vi "Initialize PID Parameters Channel Browsers.vi"(6 "Enable Gain Scheduling":bool, 8 "error in (no error)":errorcluster, 10 "Channel Browser":refnum<k24>, 11 "Item Ref in":T2 format="%.0x") -> (0 "error out":errorcluster, 2 "Refs":T1, 3 "Item Ref out":T2 format="%.0x")   [LabVIEW 2013, in "Control Addon System Explorer.lvlib"]
uses:
  Control Addon System Explorer.lvlib
  <vilib>/NI Veristand/Custom Device API/Custom Device Item Ref.ctl
  NationalInstruments.VeriStand.SystemStorageUI
  Types/PID Parameters Channel Browser Refs.ctl
  <vilib>/NI Veristand/UI Controls/Single Node Browser/Net Event Data.ctl
  <vilib>/NI Veristand/UI Controls/Single Node Browser/Net Event.ctl
  Shared/Constants.vi
  <vilib>/NI Veristand/UI Controls/Single Node Browser/NI_VS UI Single Node Browser.lvlib
  Shared/Control Addon Shared.lvlib
  <vilib>/NI VeriStand/Custom Device API/Custom Device API.lvlib
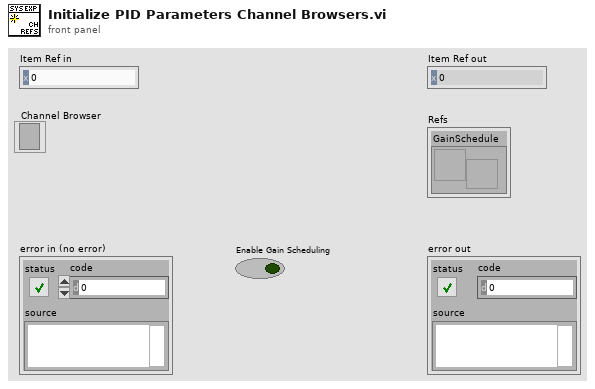
[diagram p1: front panel]
types:
  T1 = typedef "Control Addon System Explorer.lvlib/PID Parameters Channel Browser Refs.ctl" = cluster{"GainSchedule":refnum<user-event>}
  T2 = typedef "Custom Device API.lvlib/Custom Device Item Ref.ctl" = u64
  T3 = typedef "NI_VS UI Single Node Browser.lvlib/Single Node Browser Ref.ctl" = refnum<k24>
  T4 = typedef "NI_VS UI Single Node Browser.lvlib/Callback Type.ctl" = cluster{"Net Callbacks":refnum<k27>[], "Event":refnum<user-event>}
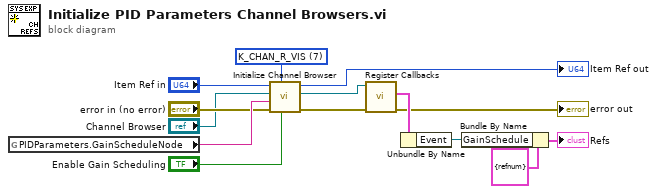
[diagram p0: block diagram]
diagram:
  w5 = u8 7 items=["K_CHAN_R", "K_CHAN_W", "K_CHAN_RW", "K_CHAN_VOLT", "K_CHAN_FAULT", "K_ALL", "K_CUSTOM", "K_CHAN_R_VIS", "K_CHAN_W_VIS", "K_CHAN_RW_VIS", "K_CHAN_VOLT_VIS", "K_CHAN_FAULT_VIS"] ("DisplayFilter")
  n1 = global read "Constants.vi" "PIDParameters.GainScheduleNode"() -> (w14:string)
  n2 = call "Initialize Channel Browser.vi"("Use Channel?"="Enable Gain Scheduling", "DisplayFilter"=w5, "error in (no error)"="error in (no error)", "NodeName"=w14, "Browser Ref"="Channel Browser", "Item Ref in"="Item Ref in") -> ("error out"=w10:errorcluster, "Browser Ref"=w9:T3, "Item Ref out"=→"Item Ref out":T2)  [unwired: 3 in]
  n3 = call <vilib>:"Register Callbacks.vi"("error in (no error)"=w10, "Single Node Browser"=w9) -> ("error out"=→"error out":errorcluster, "Callbacks"=w12:T4)  [unwired: 7 in, 1 out]
  n4 = Unbundle By Name(w12) -> ("Event"=w2:refnum<user-event>)
  n5 = Bundle By Name(cluster=T1 {"GainSchedule"=refnum}, "GainSchedule"=w2) -> (→"Refs":T1)
